vi "Laser 1 Update status data.vi"(8 "error in (no error)":errorcluster, 11 "Data":string[](array[string])) -> (0 "error out":errorcluster)   [LabVIEW 2020]
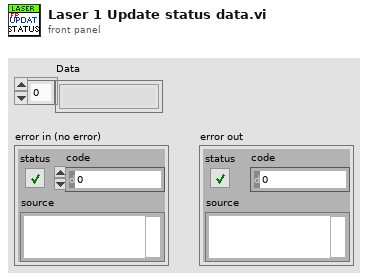
[diagram p1: front panel]
types:
  T1 = enum16{"Initialise", "Disable Controls", "Enable Controls", "Update Connection Info", "Update Laser Warning", "Update Laser status", "Update Laser Wav.", "Update prechiper settings", "Update Laser Note", "Update Shutter Status"}
  T2 = enum16{"Initialise", "Disable Controls", "Enable Controls", "Update Connection Info", "Update Laser Warning", "Update Laser status", "Update Laser Wav.", "Update prechiper settings", "Update Laser Note"}
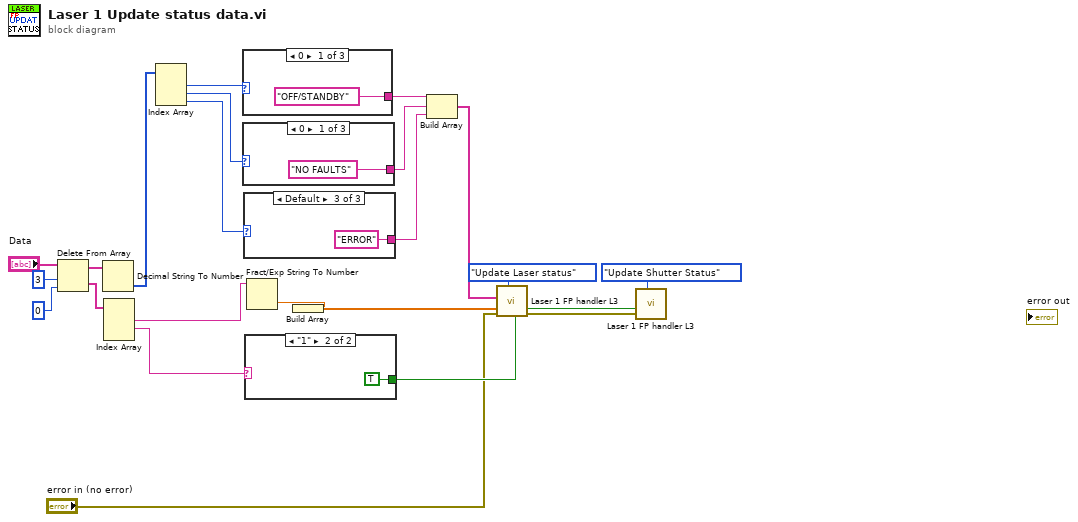
[diagram p0: block diagram]
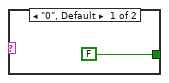
[diagram p2: hidden frame]
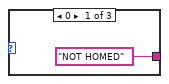
[diagram p3: hidden frame]
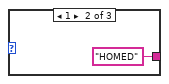
[diagram p4: hidden frame]
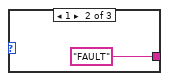
[diagram p5: hidden frame]
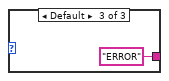
[diagram p6: hidden frame]
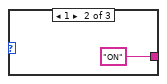
[diagram p7: hidden frame]
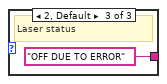
[diagram p8: hidden frame]
diagram:
  n1 = Delete From Array(array="Data", length=3, index=0) -> (deleted portion=w11:string[], array with subset deleted=w10:string[])
  n2 = Decimal String To Number(string=w10) -> (number=w1:i32[])  [unwired: 2 in, 1 out]
  n3 = Index Array(array=w11) -> (element #1=w12:string, element #2=w19:string)  [unwired: 3 in, 1 out]
  n4 = Index Array(array=w1) -> (element #1=w2:i32, element #2=w3:i32, element #3=w6:i32)  [unwired: 3 in]
  n5 = case shown="0" w2 {
    tunnel: ["OFF/STANDBY" "ON" "OFF DUE TO ERROR"] -> w13
    frame 0 {
    }
    frame 1 {
    }
    frame 2, Default {
      # "Laser status"
    }
  }
  n6 = case shown="0" w3 {
    tunnel: ["NO FAULTS" "FAULT" "ERROR"] -> w14
    frame 0 {
    }
    frame 1 {
    }
    frame Default {
    }
  }
  n7 = case shown="Default" w6 {
    tunnel: ["NOT HOMED" "HOMED" "ERROR"] -> w15
    frame 0 {
    }
    frame 1 {
    }
    frame Default {
    }
  }
  n8 = case shown="\"1\"" w19 {
    tunnel: [FALSE TRUE] -> w21
    frame "0", Default {
    }
    frame "1" {
    }
  }
  n9 = Fract/Exp String To Number(string=w12) -> (number=w17:dbl)  [unwired: 3 in, 1 out]
  n10 = Build Array(w17) -> (w18:dbl[])
  n11 = Build Array(w13, w14, w15) -> (w16:string[])
  n12 = call "Laser 1 FP handler L3.vi"("Numeric"=w18, "FP Ops"=T2."Update Laser status", "Error in"="error in (no error)", "I/p string(s)"=w16) -> ("Error out"=w22:errorcluster)  [unwired: 5 in, 2 out]
  n13 = call "Laser 1 FP handler L3.vi"("FP Ops"=T1."Update Shutter Status", "Error in"=w22, "Boolean"=w21) -> ()  [unwired: 6 in, 3 out]
